vi "GeneralInfo.vi"(7 "Mode":T1, 8 "error in (no error)":errorcluster, 9 "AcquisitionStart":T2, 10 "ChannelInfo in":T4[](array[typedef]), 11 "OXY_SCPI Reseource In":refnum<visa-resource-name>) -> (0 "error out":errorcluster, 1 "AcquisitionStart out":T2, 2 "ChannelInfo out":T4[](array[typedef]))   [LabVIEW 2020, in "OXYGEN_Datastream.lvlib"]
uses:
  OXYGEN_Datastream.lvlib
  TypeDefs/AcqInfo_AcquisitionStart.ctl
  TypeDefs/AcqInfo_AcquisitionStart_nanoseconds.ctl
  TypeDefs/ChannelInfo.ctl
  TypeDefs/ChannelInfo_Scaling.ctl
  TypeDefs/FGV_enum_GeneralInfo.ctl
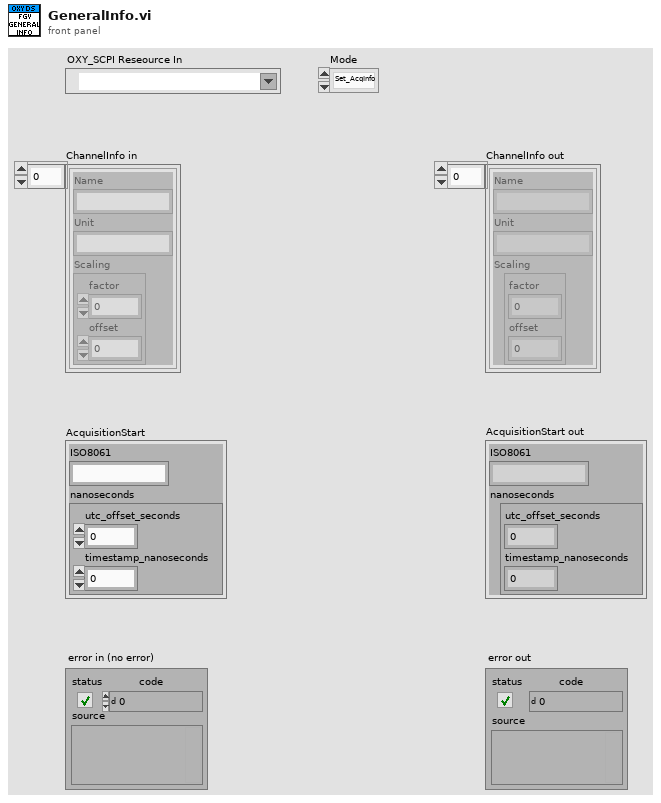
[diagram p1: front panel]
types:
  T1 = typedef "OXYGEN_Datastream.lvlib/FGV_enum_GeneralInfo.ctl" = enum16{"Set_AcqInfo", "Set_ChInfo", "Get"}
  T2 = typedef "OXYGEN_Datastream.lvlib/AcqInfo_AcquisitionStart.ctl" = cluster{"ISO8061":string, "nanoseconds":T3}
  T3 = typedef "OXYGEN_Datastream.lvlib/AcqInfo_AcquisitionStart_nanoseconds.ctl" = cluster{"utc_offset_seconds":i64, "timestamp_nanoseconds":i64}
  T4 = typedef "OXYGEN_Datastream.lvlib/ChannelInfo.ctl" = cluster{"Name":string, "Unit":string, "Scaling":T5}
  T5 = typedef "OXYGEN_Datastream.lvlib/ChannelInfo_Scaling.ctl" = cluster{"factor":dbl, "offset":dbl}
  T6 = cluster{"Id":i32, "ChannelInfo in":T4[], "AcquisitionStart":T2}
  T7 = cluster{"Id":i32, "ChannelInfo in":T4[], "AcquisitionStart":T2}[]
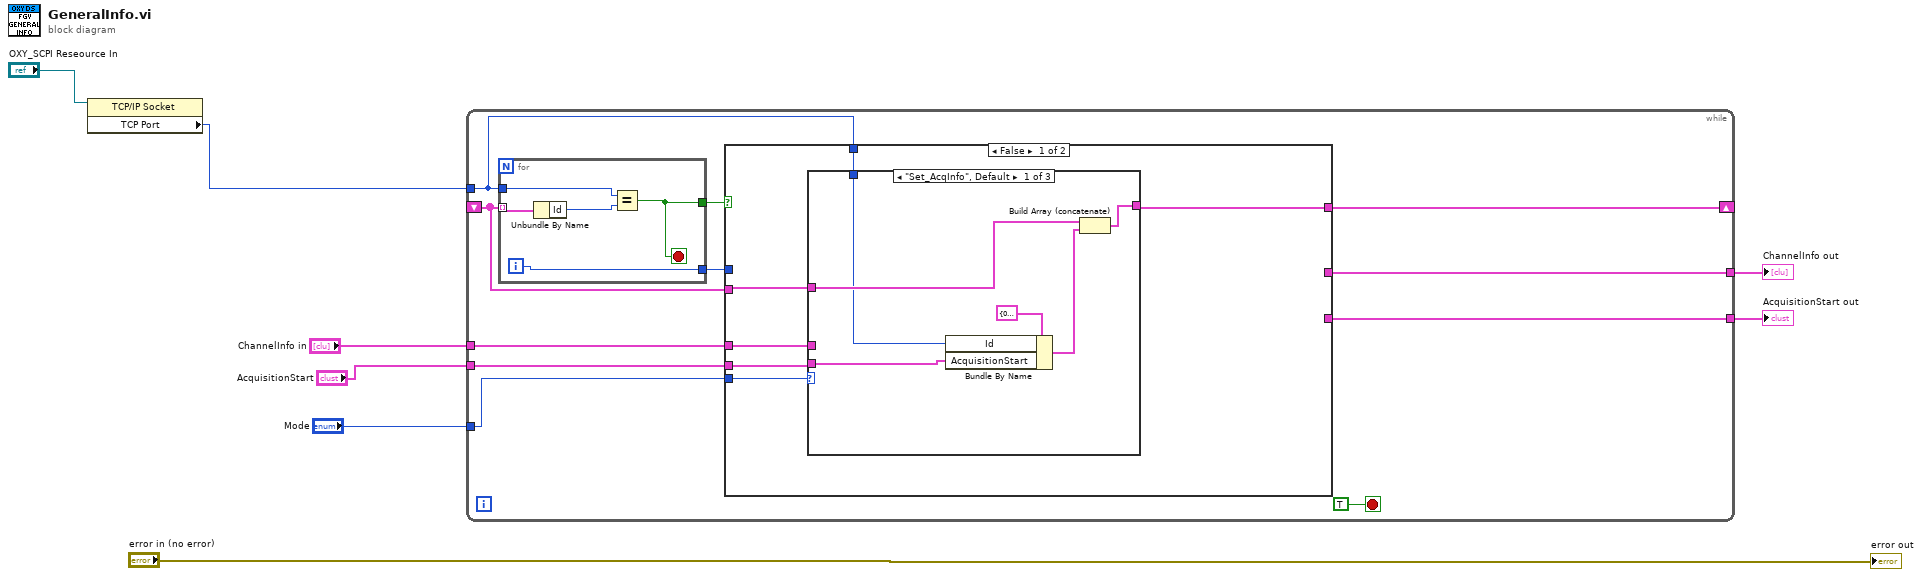
[diagram p0: block diagram]
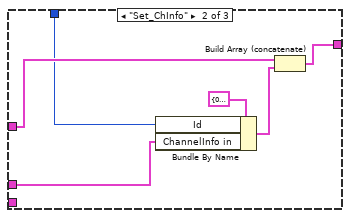
[diagram p2: hidden frame]
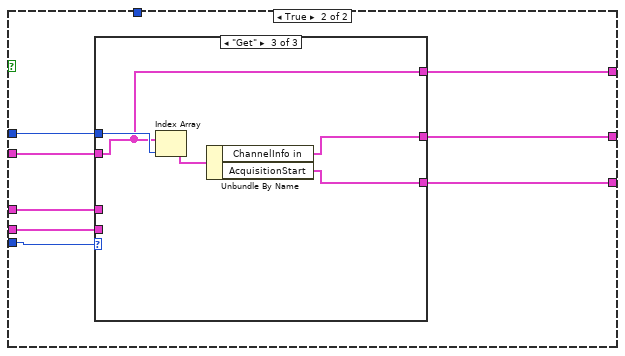
[diagram p4: hidden frame]
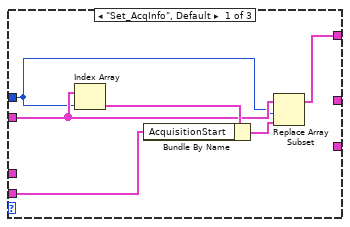
[diagram p5: hidden frame]
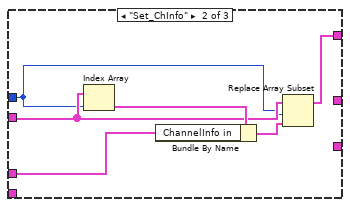
[diagram p6: hidden frame]
diagram:
  n1 = property class="TCP/IP Socket"(reference="OXY_SCPI Reseource In") -> ("TCP Port"=w5:u16)  [unwired: 1 in, 2 out]
  n2 = while {
    tunnel: "Mode" -> [w11]
    shift-right: [w14] -> _
    shift-left: _ -> [w17]
    tunnel: w5 -> [w9]
    tunnel: "AcquisitionStart" -> [w15]
    tunnel: [w13] -> w3
    tunnel: [w12] -> w2
    tunnel: "ChannelInfo in" -> [w10]
    stop <- TRUE stop-if-true
    n3 = for {
      tunnel: w17 -> [w68] mode=indexing
      tunnel: w9 -> [w64]
      tunnel: [w66] -> w18
      tunnel: [w65] -> w16
      i -> [w65]
      stop <- w66 stop-if-true
      n4 = Unbundle By Name(w68) -> ("Id"=w67:i32)
      n5 = Equal?(x=w64, y=w67) -> (x = y?=w66:bool)
    }
    n6 = case shown="False" w18 {
      tunnel: w17 -> [w24 w46]
      tunnel: w16 -> [_ w45]
      tunnel: w15 -> [w23 w44]
      tunnel: [w25 w43] -> w14
      tunnel: [_ w42] -> w13
      tunnel: [_ w41] -> w12
      tunnel: w11 -> [w22 w40]
      tunnel: w10 -> [w21 w39]
      tunnel: w9 -> [w20 _]
      frame False {
        n7 = case shown="\"Set_AcqInfo\", Default" w22 {
          tunnel: w24 -> [w29 w35 w38]
          tunnel: w23 -> [w31 _ _]
          tunnel: [w30 w34 w38] -> w25
          tunnel: w21 -> [_ w36 _]
          tunnel: w20 -> [w26 w32 _]
          frame "Set_AcqInfo", Default {
            n8 = Bundle By Name(cluster=T6 {"Id"=0, "ChannelInfo in"=[{"Name"="AI 1/I1 Sim", "Unit"="V", "Scaling"={"factor"=1.1920929665620903e-06, "offset"=0.0}}, {"Name"="AI 1/I2 Sim", "Unit"="V", "Scaling"={"factor"=1.1920929665620903e-06, "offset"=0.0}}], "AcquisitionStart"={"ISO8061"="", "nanoseconds"={"utc_offset_seconds"=0, "timestamp_nanoseconds"=0}}}, "Id"=w26, "AcquisitionStart"=w31) -> (w28:T6)
            n9 = Build Array (concatenate)(w29, w28) -> (w30:T7)
          }
          frame "Set_ChInfo" {
            n10 = Bundle By Name(cluster=T6 {"Id"=0, "ChannelInfo in"=[{"Name"="AI 1/I1 Sim", "Unit"="V", "Scaling"={"factor"=1.1920929665620903e-06, "offset"=0.0}}, {"Name"="AI 1/I2 Sim", "Unit"="V", "Scaling"={"factor"=1.1920929665620903e-06, "offset"=0.0}}], "AcquisitionStart"={"ISO8061"="", "nanoseconds"={"utc_offset_seconds"=0, "timestamp_nanoseconds"=0}}}, "Id"=w32, "ChannelInfo in"=w36) -> (w37:T6)
            n11 = Build Array (concatenate)(w35, w37) -> (w34:T7)
          }
          frame "Get" {
          }
        }
      }
      frame True {
        n12 = case shown="\"Get\"" w40 {
          tunnel: w46 -> [w49 w56 w59]
          tunnel: w45 -> [w48 w55 w63]
          tunnel: w44 -> [w51 _ _]
          tunnel: [w47 w54 w59] -> w43
          tunnel: [_ _ w61] -> w42
          tunnel: [_ _ w60] -> w41
          tunnel: w39 -> [_ w53 _]
          frame "Set_AcqInfo", Default {
            n13 = Index Array(array=w49, index=w48) -> (element=w52:T6)
            n14 = Bundle By Name(cluster=w52, "AcquisitionStart"=w51) -> (w50:T6)
            n15 = Replace Array Subset(array=w49, new element=w50, index=w48) -> (w47:T7)
          }
          frame "Set_ChInfo" {
            n16 = Index Array(array=w56, index=w55) -> (element=w58:T6)
            n17 = Bundle By Name(cluster=w58, "ChannelInfo in"=w53) -> (w57:T6)
            n18 = Replace Array Subset(array=w56, new element=w57, index=w55) -> (w54:T7)
          }
          frame "Get" {
            n19 = Index Array(array=w59, index=w63) -> (element=w62:T6)
            n20 = Unbundle By Name(w62) -> ("ChannelInfo in"=w61:T4[], "AcquisitionStart"=w60:T2)
          }
        }
      }
    }
  }
  "ChannelInfo out" <- w3
  "AcquisitionStart out" <- w2
  "error out" <- "error in (no error)"
